vi "NML SCM IPS unpersistence.vi"(3 "Input Cluster":T1 {"MaxLambdaCurrent [A]" format="%.2f"; "LambdaRates [A/min]" format="%.5e"; "MaxNormalCurrent [A]" format="%.2f"; "StabilitySetting [%]" format="%.2f"; "FieldCurrentRatio [T/A]" format="%.2f"; "SwitchWaitTime [s]" format="%.2f"; "SwitchHtrCurrent [mA]" format="%.2f"; "TrainRates [A/min]" format="%.5e"; "NormalRates [A/min]" format="%.5e"; "Breakpts [A]" format="%.5e"}, 5 "VISA session":refnum<visa-resource-name>="GPIB0::22::INSTR") -> (0 "Persistence Out":bool, 1 "String":string, 2 "dup VISA session":refnum<visa-resource-name>)   [LabVIEW 2019]
uses:
  Instance           6 33Saved   NML SCM IPS unpersistance .vi
panel:
  out "Persistence In":bool
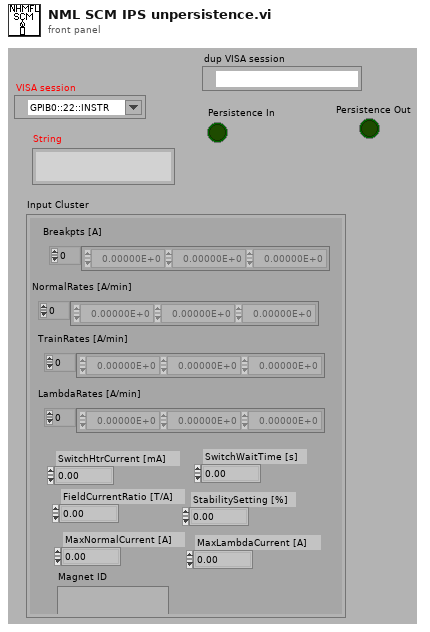
[diagram p1: front panel]
types:
  T1 = cluster{"Breakpts [A]":dbl[], "NormalRates [A/min]":dbl[], "TrainRates [A/min]":dbl[], "SwitchHtrCurrent [mA]":dbl, "SwitchWaitTime [s]":dbl, "FieldCurrentRatio [T/A]":dbl, "StabilitySetting [%]":dbl, "MaxNormalCurrent [A]":dbl, "Magnet ID":string, "LambdaRates [A/min]":dbl[], "MaxLambdaCurrent [A]":dbl}
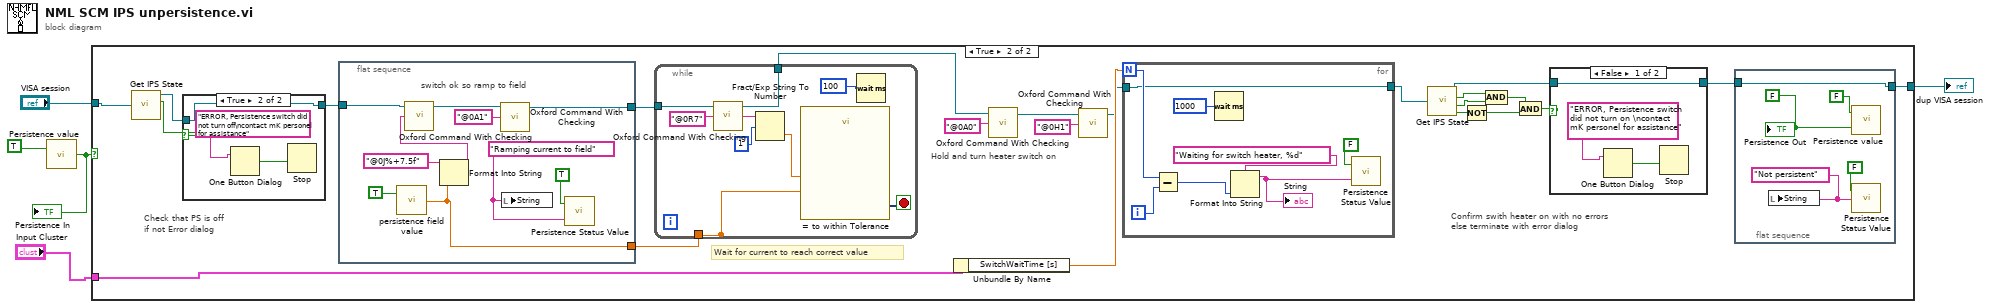
[diagram p0: block diagram]
diagram:
  n1 = call "Persistence value.vi"("Persistence In"=TRUE ("Read/Write")) -> ("Persistence Out"=w3:bool)  [unwired: 1 in]
  "Persistence In" <- w3
  n2 = case shown="True" w3 {
    tunnel: "VISA session" -> [w6 w29]
    tunnel: "Input Cluster" -> [_ w16]
    tunnel: [w6 w7] -> w1
    frame False {
      # "Not persistent so ignore"
    }
    frame True {
      # "Wait for current to reach correct value"
      # "Confirm swith heater on with no errors\nelse terminate with error dialog"
      # "Hold and turn heater switch on"
      # "Check that PS is off \nif not Error dialog"
      n3 = call "Get IPS State.vi"("VISA session"=w29) -> ("dup VISA session"=w26:refnum<visa-resource-name>, "Switch Heater"=w27:bool)  [unwired: 1 in, 3 out]
      n4 = case shown="True" w27 {
        tunnel: [w66 w67] -> w28
        tunnel: w26 -> [w66 w67]
        frame False {
        }
        frame True {
          n5 = One Button Dialog(message="ERROR, Persistence switch did not turn off\ncontact mK personel for assistance") -> (true=w68:bool)  [unwired: 1 in]
          n6 = Stop(stop? (T)=w68) -> ()
        }
      }
      n7 = flat-sequence {
        tunnel: w28 -> [w47]
        tunnel: [w44] -> w22
        tunnel: [w43] -> w21
        frame #0 {
          w52 = "Ramping current to field" ("String")
          # "switch ok so ramp to field"
          n8 = call "persistence field value.vi"("Read/Write this vi"=TRUE) -> ("Persistent Field Out"=w43:dbl)  [unwired: 1 in]
          n9 = Format Into String(format string="@0J%+7.5f" ("Command String"), w43) -> (resulting string=w48:string)  [unwired: 2 in, 1 out]
          n10 = call "Oxford Command With Checking.vi"("Command"=w48, "VISA session"=w47) -> ("dup VISA session"=w46:refnum<visa-resource-name>)  [unwired: 1 in, 2 out]
          n11 = call "Oxford Command With Checking.vi"("Command"="@0A1", "VISA session"=w46) -> ("dup VISA session"=w44:refnum<visa-resource-name>)  [unwired: 1 in, 2 out]
          n12 = local write "String"(w52) -> ()
          n13 = call "Persistence Status Value.vi"("Persistence Status In"=w52, "Read/Write this vi"=TRUE) -> ()  [unwired: 1 out]
        }
      }
      n14 = while {
        tunnel: w22 -> [w64]
        tunnel: [w59] -> _
        tunnel: w21 -> [w59]
        tunnel: [w57] -> w19
        stop <- w58 stop-if-true
        n15 = call "Oxford Command With Checking.vi"("Command"="@0R7", "VISA session"=w64) -> ("String Read"=w62:string, "dup VISA session"=w57:refnum<visa-resource-name>)  [unwired: 1 in, 1 out]
        n16 = Fract/Exp String To Number(string=w62, offset=1) -> (number=w60:dbl)  [unwired: 2 in, 1 out]
        n17 = call "= to within Tolerance"("Constant Value to Compare Against"=w59, "Operand 1"=w60) -> ("Result"=w58:dynamicdata)  [unwired: 8 in, 1 out]
        n18 = Wait (ms)(milliseconds to wait=u32 100) -> ()  [unwired: 1 out]
      }
      n19 = Unbundle By Name(w16) -> ("SwitchWaitTime [s]"=w15:dbl)
      n20 = call "Oxford Command With Checking.vi"("Command"="@0A0", "VISA session"=w19) -> ("dup VISA session"=w17:refnum<visa-resource-name>)  [unwired: 1 in, 2 out]
      n21 = call "Oxford Command With Checking.vi"("Command"="@0H1", "VISA session"=w17) -> ("dup VISA session"=w14:refnum<visa-resource-name>)  [unwired: 1 in, 2 out]
      n22 = for {
        N: w15 -> [w39]
        tunnel: w14 -> [w35]
        tunnel: [w35] -> w8
        i -> [w40]
        n23 = Subtract(x=w39, y=w40) -> (x-y=w38:i32)
        n24 = Wait (ms)(milliseconds to wait=u32 1000) -> ()  [unwired: 1 out]
        n25 = Format Into String(format string="Waiting for switch heater, %d", w38) -> (resulting string=w37:string)  [unwired: 2 in, 1 out]
        "String" <- w37
        n26 = call "Persistence Status Value.vi"("Persistence Status In"=w37, "Read/Write this vi"=FALSE) -> ()  [unwired: 1 out]
      }
      n27 = call "Get IPS State.vi"("VISA session"=w8) -> ("dup VISA session"=w13:refnum<visa-resource-name>, "Switch Heater"=w11:bool, "Switch heater \nconfirmed"=w10:bool, "Switch Heater Error"=w9:bool)  [unwired: 1 in, 1 out]
      n28 = Not(x=w9) -> (.not. x?=w24:bool)
      n29 = And(x=w11, y=w10) -> (x .and. y?=w25:bool)
      n30 = And(x=w25, y=w24) -> (x .and. y?=w23:bool)
      n31 = case shown="False" w23 {
        tunnel: w13 -> [w53 w56]
        tunnel: [w53 w56] -> w12
        frame False {
          n32 = One Button Dialog(message="ERROR, Persistence switch did not turn on \ncontact mK personel for assistance") -> (true=w54:bool)  [unwired: 1 in]
          n33 = Stop(stop? (T)=w54) -> ()
        }
        frame True {
        }
      }
      n34 = flat-sequence {
        tunnel: w12 -> [w30]
        tunnel: [w30] -> w7
        frame #0 {
          w34 = "Not persistent" ("String")
          w33 = FALSE
          n35 = local write "String"(w34) -> ()
          n36 = call "Persistence value.vi"("Persistence In"=w33, "Read/Write this vi"=FALSE) -> ()  [unwired: 1 out]
          n37 = call "Persistence Status Value.vi"("Persistence Status In"=w34, "Read/Write this vi"=FALSE) -> ()  [unwired: 1 out]
          "Persistence Out" <- w33
        }
      }
    }
  }
  "dup VISA session" <- w1
